vi "Main.vi"(8 "error in (no error)":errorcluster, 11 "Process in":refnum<class "Process.lvclass">) -> (0 "error out":errorcluster, 3 "Process out":refnum<class "Process.lvclass">)   [LabVIEW 2019, in "TimingDRV Engine.lvlib" / "Process.lvclass"]
uses:
  Process.lvclass
  Process.lvclass/Process.ctl
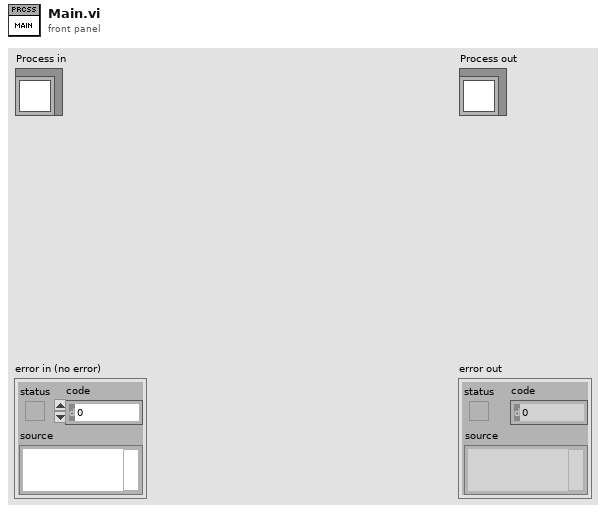
[diagram p1: front panel]
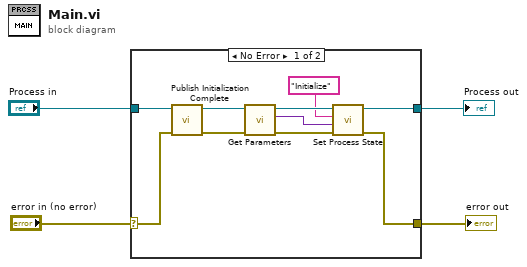
[diagram p0: block diagram]
diagram:
  n1 = case shown="No Error" "error in (no error)" {
    selector: "error in (no error)" -> [w12 w15]
    tunnel: [w10 w15] -> w3
    tunnel: [w11 w14] -> w1
    tunnel: "Process in" -> [w13 w14]
    frame No Error {
      n2 = call "Publish Initialization Complete.vi"("error in (no error)"=w12, "Process in"=w13) -> ("error out"=w6:errorcluster, "Process out"=w9:refnum<class "Process.lvclass">)  [unwired: 8 in]
      n3 = call "Get Parameters.vi"("Process in"=w9) -> ("Parameters"=w7:variant, "Process out"=w8:refnum<class "Process.lvclass">)  [unwired: 9 in]
      n4 = call "Set Process State.vi"("error in (no error)"=w6, "Payload"=w7, "Command"="Initialize", "Process in"=w8) -> ("error out"=w10:errorcluster, "Process out"=w11:refnum<class "Process.lvclass">)  [unwired: 6 in]
    }
    frame Error {
    }
  }
  "error out" <- w3
  "Process out" <- w1
